vi "tm_getfunctionlist.vi"(8 "error in (no error)":errorcluster, 11 "Handle in":u32) -> (0 "error out":errorcluster, 2 "Function List":T1(array[cluster]), 3 "Handle out":u32)   [LabVIEW 2011]
uses:
  tmcamcon.dll
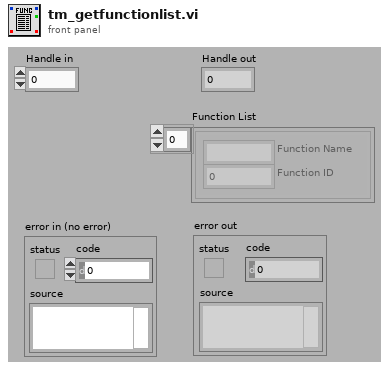
[diagram p1: front panel]
types:
  T1 = cluster{"Function Name":string, "Function ID":dbl}[]
  T2 = cluster{"Property Name":string, "Property ID":dbl}[]
  T3 = cluster{"Property Name":string, "Property ID":dbl}
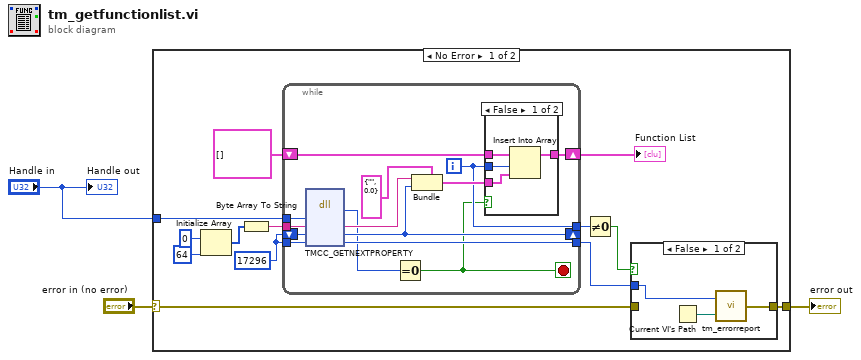
[diagram p0: block diagram]
diagram:
  n1 = case shown="No Error" "error in (no error)" {
    selector: "error in (no error)" -> [w7 w40]
    tunnel: [w4 w40] -> w2
    tunnel: "Handle in" -> [w8 _]
    frame No Error {
      w14 = 17296
      n2 = Initialize Array(u8 0 ("element"), 64 ("dimension size")) -> (w9:u8[])
      n3 = Byte Array To String(unsigned byte array=w9) -> (string=w12:string)
      n4 = while {
        shift-right: [w33] -> w15
        shift-left: T2 [] ("Array") -> [w34]
        tunnel: w14 -> [w29]
        tunnel: [w28] -> w6
        tunnel: [w26] -> w13
        tunnel: w12 -> [w25]
        tunnel: w8 -> [w24]
        shift-right: [w27] -> _
        shift-left: w14 -> [w30]
        i -> [w26]
        stop <- w22 stop-if-true
        n5 = dll-call lib="tmcamcon.dll" fn="TMCC_GETNEXTPROPERTY"("HDCAM"=w24, "name"=w25, "prop"=w30, "Erval"=w29) -> ("return type"=w21:u32, "name"=w31:string, "prop"=w27:i32, "Erval"=w28:i32)  [unwired: 4 in, 2 out]
        n6 = Equal To 0?(x=w21) -> (x = 0?=w22:bool)
        n7 = Bundle(cluster=T3 {"Property Name"="", "Property ID"=0.0} ("new element/subarray"), "Property Name"=w31, "Property ID"=w27) -> (w32:T3)
        n8 = case shown="False" w22 {
          tunnel: w34 -> [w38 w39]
          tunnel: [w37 w39] -> w33
          tunnel: w26 -> [w36 _]
          tunnel: w32 -> [w35 _]
          frame False {
            n9 = Insert Into Array(array=w38, index=w36, new element=w35) -> (w37:T2)
          }
          frame True {
          }
        }
      }
      "Function List" <- w15
      n10 = Not Equal To 0?(x=w13) -> (x != 0?=w5:bool)
      n11 = case shown="False" w5 {
        tunnel: w7 -> [_ w20]
        tunnel: [w18 w20] -> w4
        tunnel: w6 -> [w17 _]
        frame False {
          n12 = Current VI's Path() -> (path=w19:path)
          n13 = call <userlib>:"tm_errorreport.vi"("Source"=w19, "Error"=w17) -> ("error out"=w18:errorcluster)
        }
        frame True {
        }
      }
    }
    frame Error {
    }
  }
  "error out" <- w2
  "Handle out" <- "Handle in"
